vi "Caraya_Dummy.vi"() -> ()   [LabVIEW 2020]
uses:
  PPL/Caraya.lvlibp/1abvi3w/vi.lib/addons/_JKI Toolkits/Caraya/classes/Assert/Assert Equal Value_Variant.vi
  PPL/Caraya.lvlibp/1abvi3w/vi.lib/addons/_JKI Toolkits/Caraya/classes/Test/Test.lvclass
  PPL/Caraya.lvlibp/1abvi3w/vi.lib/addons/_JKI Toolkits/Caraya/classes/Assert/Assert.lvclass
panel:
  out "error out":errorcluster
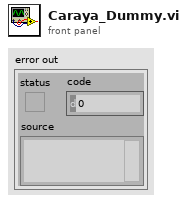
[diagram p1: front panel]
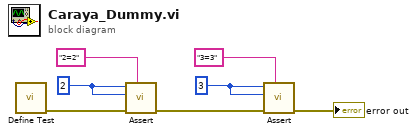
[diagram p0: block diagram]
diagram:
  w4 = 3
  w7 = 2
  n1 = call "Define Test.vi"() -> ("error out"=w5:errorcluster)  [unwired: 11 in]
  n2 = call-poly "Assert.vi"("Label"="2=2", "error in (no error)"=w5, "Y"=w7, "X"=w7) -> ("error out"=w1:errorcluster)  [unwired: 7 in]
  n3 = call-poly "Assert.vi"("Label"="3=3", "error in (no error)"=w1, "Y"=w4, "X"=w4) -> ("error out"=→"error out":errorcluster)  [unwired: 7 in]
